vi "CV ICCD Data Plot.vi"(8 "Error In":errorcluster, 9 "ICCD Parameter Set":T2, 10 "Abscissa":enum32{"I-", "<I>"}(radio), 11 "Analysis Data Folder":path) -> (0 "Error Out":errorcluster, 1 "File Name":string, 2 "I Range":cluster{"Minimum":dbl, "Maximum":dbl}, 3 "Plot":T1)   [LabVIEW 2021, in "AlliGator Camera Noise Influence on Lifetime.lvlib"]
uses:
  AlliGator Camera Noise Influence on Lifetime.lvlib
  ICCD Parameter Set.ctl
  Graphs/XY Graph/XY Graph Plot Data.ctl
  Files/Files.lvlib
  b667337d-681e-4974-8c7b-9b0992625a42.vi
  Graphs/XY Graph/XY Graph Add-Ons.lvlib
panel:
  out "Column Headers":string
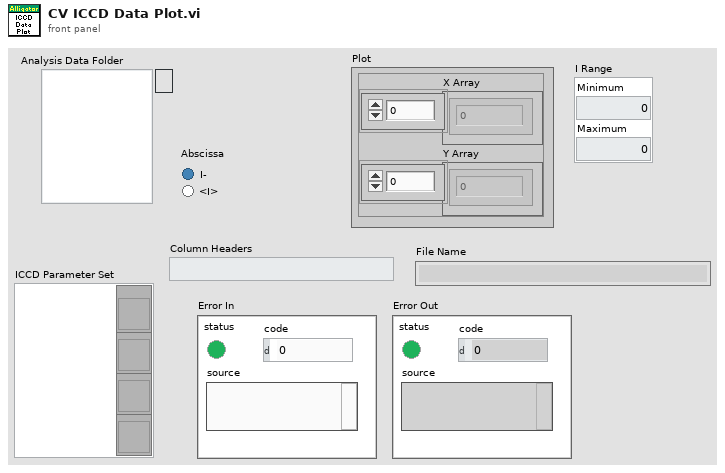
[diagram p1: front panel]
types:
  T1 = typedef "XY Graph Add-Ons.lvlib/XY Graph Plot Data.ctl" = cluster{"X Array":dbl[], "Y Array":dbl[]}
  T2 = typedef "AlliGator Camera Noise Influence on Lifetime.lvlib/ICCD Parameter Set.ctl" = cluster{"Binning":refnum<vi>, "Exposure (ms)":refnum<vi>, "Laser Power (mW)":refnum<vi>, "MCP Voltage (V)":refnum<vi>}
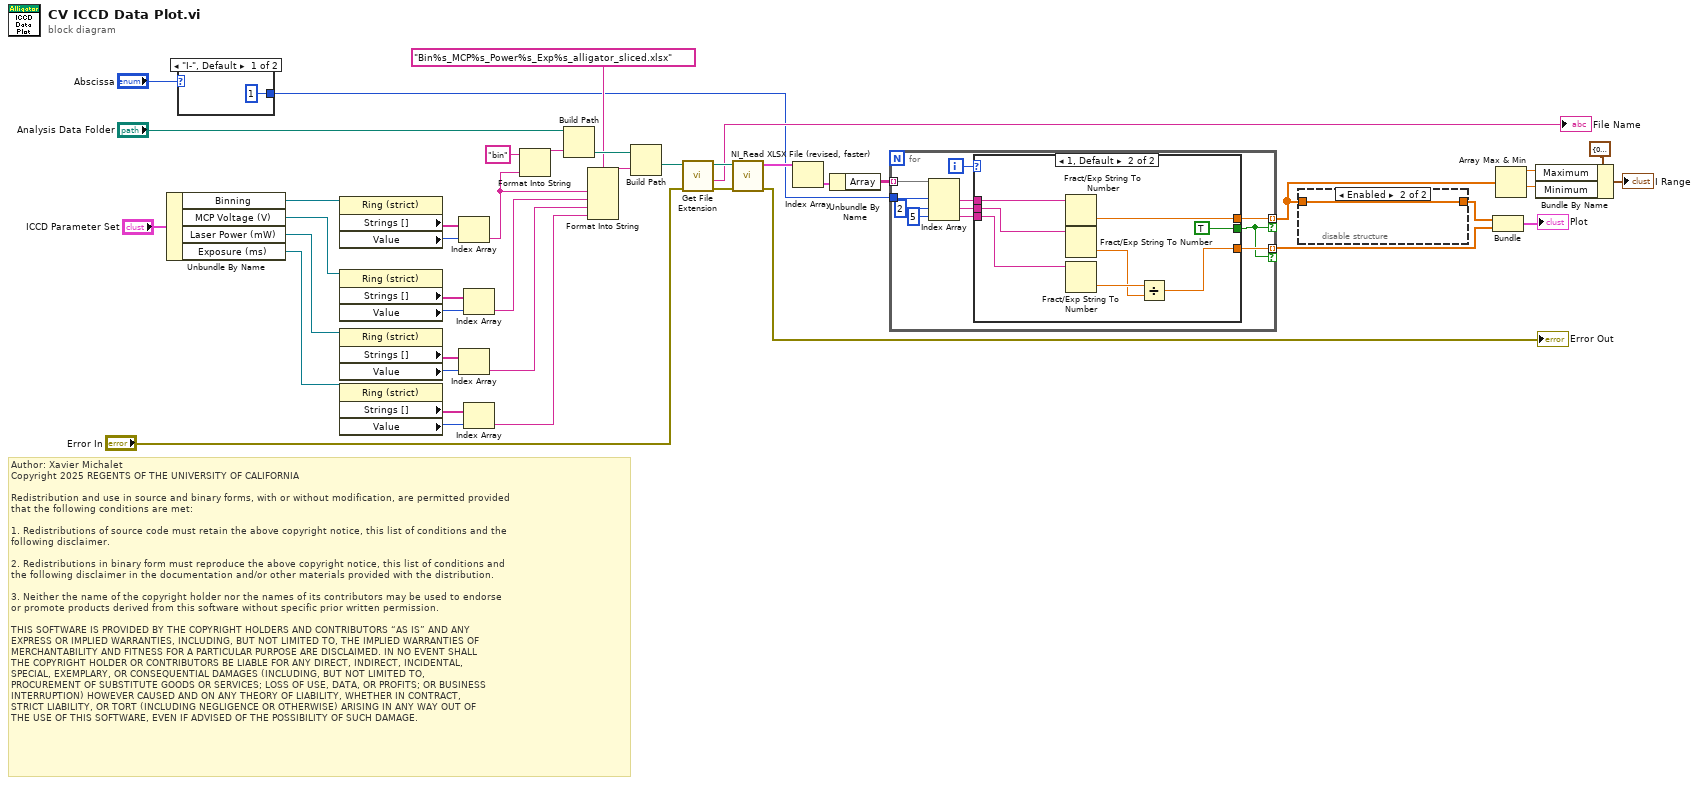
[diagram p0: block diagram]
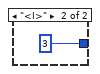
[diagram p2: hidden frame]
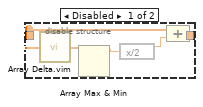
[diagram p3: hidden frame]
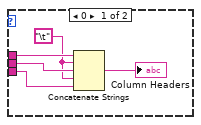
[diagram p4: hidden frame]
diagram:
  # "Author: Xavier Michalet\nCopyright 2025 REGENTS OF THE UNIVERSITY OF CALIFORNIA\n\nRedistribution and use in source and binary forms, with or without modification, are permitted provided\nthat the following conditions are met:\n\n1. Redistributions of source code must retain the above copyright notice, this list of conditions and the\nfollowing disclaimer.\n\n2. Redistributions in binary form must reproduce the above copyright notice, this list of conditions and\nthe following disclaimer in the documentation and/or other materials provided with the distribution.\n\n3. Neither the name of the copyright holder nor the names of its contributors may be used to endorse \nor promote products derived from this software without specific prior written permission.\n\nTHIS SOFTWARE IS PROVIDED BY THE COPYRIGHT HOLDERS AND CONTRIBUTORS “AS IS” AND ANY \nEXPRESS OR IMPLIED WARRANTIES, INCLUDING, BUT NOT LIMITED TO, THE IMPLIED WARRANTIES OF\nMERCHANTABILITY AND FITNESS FOR A PARTICULAR PURPOSE ARE DISCLAIMED. IN NO EVENT SHALL\nTHE COPYRIGHT HOLDER OR CONTRIBUTORS BE LIABLE FOR ANY DIRECT, INDIRECT, INCIDENTAL, \nSPECIAL, EXEMPLARY, OR CONSEQUENTIAL DAMAGES (INCLUDING, BUT NOT LIMITED TO, \nPROCUREMENT OF SUBSTITUTE GOODS OR SERVICES; LOSS OF USE, DATA, OR PROFITS; OR BUSINESS\nINTERRUPTION) HOWEVER CAUSED AND ON ANY THEORY OF LIABILITY, WHETHER IN CONTRACT, \nSTRICT LIABILITY, OR TORT (INCLUDING NEGLIGENCE OR OTHERWISE) ARISING IN ANY WAY OUT OF\nTHE USE OF THIS SOFTWARE, EVEN IF ADVISED OF THE POSSIBILITY OF SUCH DAMAGE."
  n1 = Unbundle By Name("ICCD Parameter Set") -> ("Binning"=w42:refnum<vi>, "MCP Voltage (V)"=w37:refnum<vi>, "Laser Power (mW)"=w32:refnum<vi>, "Exposure (ms)"=w31:refnum<vi>)
  n2 = case shown="\"I-\", Default" "Abscissa" {
    tunnel: [1 ("index") 3 ("index")] -> w1
    frame "I-", Default {
    }
    frame "<I>" {
    }
  }
  n3 = property class="Ring (strict)"(reference=w42) -> ("Strings []"=w41:string[], "Value"=w40:i32)  [unwired: 1 in, 2 out]
  n4 = property class="Ring (strict)"(reference=w37) -> ("Strings []"=w39:string[], "Value"=w38:i32)  [unwired: 1 in, 2 out]
  n5 = property class="Ring (strict)"(reference=w32) -> ("Strings []"=w33:string[], "Value"=w34:i32)  [unwired: 1 in, 2 out]
  n6 = property class="Ring (strict)"(reference=w31) -> ("Strings []"=w35:string[], "Value"=w36:i32)  [unwired: 1 in, 2 out]
  n7 = Index Array(array=w41, index=w40) -> (element=w14:string)
  n8 = Index Array(array=w33, index=w34) -> (element=w23:string)
  n9 = Index Array(array=w39, index=w38) -> (element=w15:string)
  n10 = Index Array(array=w35, index=w36) -> (element=w22:string)
  n11 = Format Into String(initial string="bin", w14) -> (resulting string=w27:string)  [unwired: 2 in, 1 out]
  n12 = Build Path(base path="Analysis Data Folder", name or relative path=w27) -> (appended path=w26:path)
  n13 = Format Into String(format string="Bin%s_MCP%s_Power%s_Exp%s_alligator_sliced.xlsx", w14, w15, w23, w22) -> (resulting string=w25:string)  [unwired: 2 in, 1 out]
  n14 = Build Path(base path=w26, name or relative path=w25) -> (appended path=w13:path)
  n15 = call <vilib>:"Get File Extension.vi"("error in (no error)"="Error In", "file"=w13) -> ("error out"=w11:errorcluster, "filename without extension"=→"File Name":string, "dup file"=w10:path)  [unwired: 5 in, 2 out]
  n16 = call "NI_Read XLSX File (revised, faster).vi"("error in"=w11, "XLSX File"=w10) -> ("error out"=→"Error Out":errorcluster, "Sheet Data"=w21:cluster{"Array":string[][]}[])  [unwired: 7 in, 1 out]
  n17 = Index Array(array=w21) -> (element=w20:cluster{"Array":string[][]})  [unwired: 1 in]
  n18 = Unbundle By Name(w20) -> ("Array"=w19:string[][])
  n19 = for {
    tunnel: w19 -> [w55] mode=indexing
    tunnel: [w49] -> w4 mode=indexing if=w47
    tunnel: [w48] -> w18 mode=indexing if=w47
    tunnel: w1 -> [w45]
    i -> [w53]
    n20 = Index Array(array=w55, index #1=w45, index #2=2 ("index"), index #3=5 ("index")) -> (element #1=w52:string, element #2=w51:string, element #3=w50:string)
    n21 = case shown="1, Default" w53 {
      tunnel: w52 -> [w60 w68]
      tunnel: w51 -> [w59 w66]
      tunnel: w50 -> [w58 w65]
      tunnel: [_ w67] -> w49
      tunnel: [_ w62] -> w48
      tunnel: [_ TRUE] -> w47
      frame 0 {
        w57 = "\t"
        n22 = Concatenate Strings(w60, w57, w59, w57, w58) -> (→"Column Headers":string)
      }
      frame 1, Default {
        n23 = Fract/Exp String To Number(string=w68) -> (number=w67:dbl)  [unwired: 3 in, 1 out]
        n24 = Fract/Exp String To Number(string=w66) -> (number=w63:dbl)  [unwired: 3 in, 1 out]
        n25 = Fract/Exp String To Number(string=w65) -> (number=w64:dbl)  [unwired: 3 in, 1 out]
        n26 = Divide(x=w64, y=w63) -> (x/y=w62:dbl)
      }
    }
  }
  n27 = disable-structure shown="Enabled" {
    disable-tunnel: w4 -> [w70 w74]
    disable-tunnel: [w69 w74] -> w3
    frame Disabled {
      n28 = call "Array Delta.vim"("A"=w70) -> ("A[i+1]-A[i]"=w73:dbl[])  [unwired: 8 in]
      n29 = Array Max & Min(array=w73) -> (max value=w72:dbl)  [unwired: 3 out]
      n30 = expression code="x/2"(w72) -> (w71:dbl)
      n31 = Compound Arithmetic op=ADD(w70, w71) -> (w69:dbl[])
    }
    frame Enabled {
    }
  }
  n32 = Bundle(w3, w18) -> (→"Plot":cluster{dbl[], dbl[]})  [unwired: 1 in]
  n33 = Array Max & Min(array=w4) -> (max value=w8:dbl, min value=w7:dbl)  [unwired: 2 out]
  n34 = Bundle By Name(cluster=cluster{"Minimum":dbl, "Maximum":dbl} {"Minimum"=0.0, "Maximum"=10000.0} ("I Range"), "Maximum"=w8, "Minimum"=w7) -> (→"I Range":cluster{"Minimum":dbl, "Maximum":dbl})
